vi "SL TAGS Set Values.vi"(6 "Tag Type":T2=enum."Supervisor", 8 "error in (no error)":errorcluster, 9 "Tag Scope":T1=enum."Server", 10 "Tag Update Values":T3[](array[typedef]), 11 "EEISysLink in":refnum<class "EEISysLink.lvclass">) -> (0 "error out":errorcluster, 3 "EEISysLink out":refnum<class "EEISysLink.lvclass">)   [LabVIEW 2017, in "EEISysLink.lvclass"]
doc: "Update the tag values to match those input to this method. The scope input will indicate whether to update only the local tag instance or to update the value to the SystemLink server. Only the tags with a matching tag type will be updated. \n\nJames Tillett\nEndeavor Engineering Inc.\nwww.endeavoreng.com"
uses:
  EEISysLink.lvclass
  Controls/SL Tag Value.ctl
  Controls/SL Tag Data Type.ctl
  Controls/SL Tag Type.ctl
  Controls/SL Tag Scope.ctl
  EEISysLink.lvclass/EEISysLink.ctl
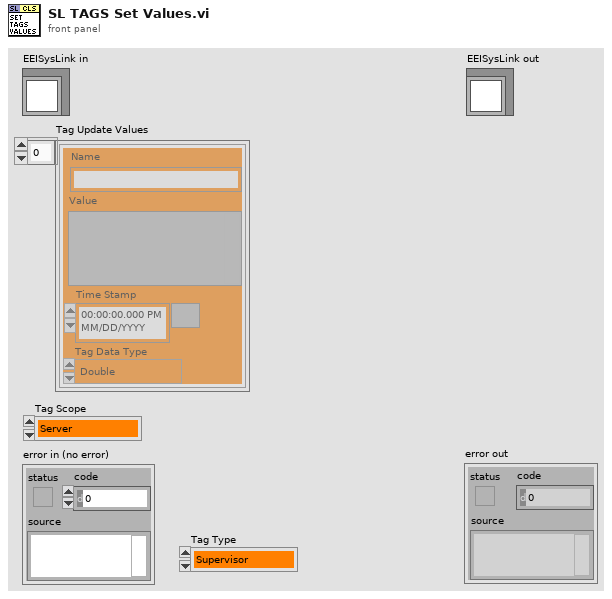
[diagram p1: front panel]
types:
  T1 = typedef "EEISysLink.lvclass/SL Tag Scope.ctl" = enum16{"Local", "Server"}
  T2 = typedef "EEISysLink.lvclass/SL Tag Type.ctl" = enum16{"All", "Supervisor", "Worker"}
  T3 = typedef "SL Tag Value.ctl" = cluster{"Value":variant, "Time Stamp":timestamp, "Tag Data Type":T4, "Name":string}
  T4 = typedef "EEISysLink.lvclass/SL Tag Data Type.ctl" = enum16{"Double", "Integer", "String", "Boolean", "Waveform"}
  T5 = typedef "EEISysLink.lvclass/SL Tag.ctl" = cluster{"Class Properties":T6, "SL Tag":refnum<class "NI Skyline Tag.lvclass">, "SystemLink Cluster":T9, "Class Value":variant}
  T6 = typedef "EEISysLink.lvclass/SL Tag Properties.ctl" = cluster{"Class Data Type":T4, "Name":string, "Description":string, "Interpolation Method":T7, "Unit of Measure":T8, "Maximum Interpolation":string, "Role":T2}
  T7 = typedef "EEISysLink.lvclass/SL Tag Interpolation Method.ctl" = enum16{"linear", "pilinear", "step"}
  T8 = typedef "EEISysLink.lvclass/SL Tag Unit of Measure.ctl" = enum16{"no units", "Second", "Hour", "Minute", "Day", "Year", "Month", "Week", "Foot", "Yard", "Meter", "Centimeter", "Inch", "Mile", "Nautical Mile", "Miles per Hour", "Meters per second", "Square meter", "Cubic meter", "Cubic centimeter", "Cubic inch", "Liter", "Gallon", "Gallons dry US", "Gallon UK", "Percent", "Revolutions per minute", "Revolution", "Degree angle", "Astronomical Unit", "Atom", "Atomic mass", "Bar", "Byte", "C (speed of light)", "Curie", "Decibel", "Electron Volt", "Ounce", "Knot", "G", "Grade", "Are", "Hectare", "Faraday", "Franklin", "Gilbert", "Erg", "Lambert", "Maxwell", "Gauss", "Electron mass", "Kilogram force", "Pound force", "Rad", "Centiradian", "Sphere", "Mach", "Fluid Ounces", "Fluid Ounces UK", "Fahrenheit", "Celsius", "Kelvin", "Rankine", "Gram", "Kilogram", "Pound", "Short/US Ton", "Long/UK ton", "Metric ton", "Mole", "Pounds per square inch", "Inches water column", "Torr", "Millitorr", "Millimeter mercury", "Inches mercury", "Bar (2)", "Atmosphere", "Pascal", "Watt", "kiloWatt", "Horsepower", "Kilowatt Hour", "British thermal units", "Millions of BTU", "Ampere", "Candela", "Radian", "Steradian", "Bit", "Hertz", "Newton", "Joule", "Coulomb", "Volt", "Farad", "Ohm", "Siemens", "Weber", "Tesla", "Henry", "Lumen", "Lux", "Becqueral", "Gray", "Sievert", "Katal", "Angstrom", "Light Year", "Parsec", "Point", "Pixel", "Dyne", "Kilogram force (2)", "Pound force (2)", "Rem", "Rutherford", "Roentgen"}
  T9 = typedef "NI Skyline Tag.lvlib/Tag Cluster.ctl" = cluster{"Path":string, "Data Type":T10, "Value":variant, "Time Stamp":timestamp}
  T10 = typedef "NI Skyline Tag.lvlib/DataType.ctl" = enum32{"Double", "Integer", "String"}
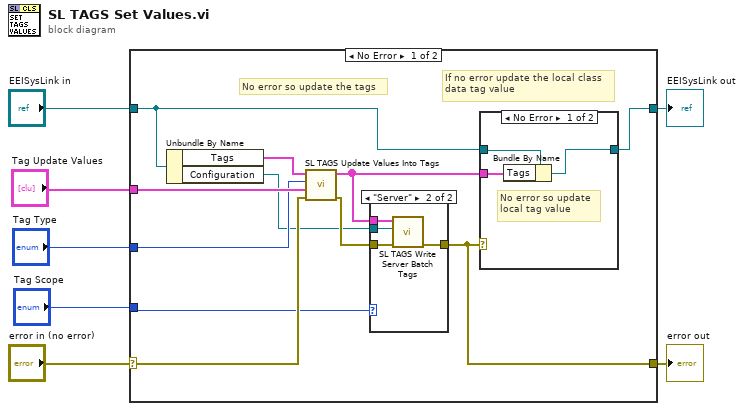
[diagram p0: block diagram]
diagram:
  n1 = case shown="No Error" "error in (no error)" {
    selector: "error in (no error)" -> [w12 w29]
    tunnel: [w16 w29] -> w6
    tunnel: [w17 w28] -> w4
    tunnel: "EEISysLink in" -> [w18 w28]
    tunnel: "Tag Update Values" -> [w14 _]
    tunnel: "Tag Type" -> [w13 _]
    tunnel: "Tag Scope" -> [w10 _]
    frame No Error {
      # "If no error update the local class\ndata tag value"
      # "No error so update the tags"
      n2 = Unbundle By Name(w18) -> ("Tags"=w15:T5[], "Configuration"=w8:refnum<class "NI Skyline Configuration.lvclass">)
      n3 = call "SL TAGS Update Values Into Tags.vi"("error in (no error)"=w12, "Tag Update Values"=w14, "Tag Type"=w13, "Tags In"=w15) -> ("error out"=w11:errorcluster, "Tags Out"=w9:T5[])  [unwired: 6 in]
      n4 = case shown="\"Server\"" w10 {
        tunnel: w9 -> [_ w21]
        tunnel: [w19 w23] -> w16
        tunnel: w11 -> [w19 w22]
        tunnel: w8 -> [_ w20]
        frame "Local", Default {
        }
        frame "Server" {
          n5 = call "SL TAGS Write Server Batch Tags.vi"("error in (no error)"=w22, "Configuration"=w20, "Tags In"=w21) -> ("error out"=w23:errorcluster)  [unwired: 7 in, 1 out]
        }
      }
      n6 = case shown="No Error" w16 {
        tunnel: w9 -> [w25 _]
        tunnel: w18 -> [w26 w27]
        tunnel: [w24 w27] -> w17
        frame No Error {
          # "No error so update\nlocal tag value"
          n7 = Bundle By Name(cluster=w26, "Tags"=w25) -> (w24:refnum<class "EEISysLink.lvclass">)
        }
        frame Error {
        }
      }
    }
    frame Error {
    }
  }
  "error out" <- w6
  "EEISysLink out" <- w4
